vi "Write.vi"(9 "Data":u8 format="%02x", 10 "Address":u16 format="%.0x", 11 "Memory in":refnum<class "Memory.lvclass">) -> (3 "Memory out":refnum<class "Memory.lvclass">)   [LabVIEW 2021, in "Memory.lvclass"]
uses:
  Memory.lvclass
  Memory.lvclass/Memory.ctl
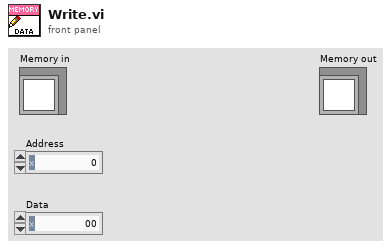
[diagram p1: front panel]
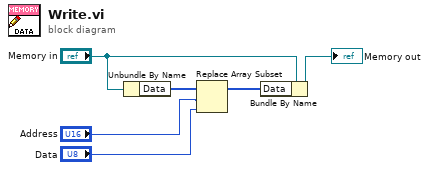
[diagram p0: block diagram]
diagram:
  n1 = Unbundle By Name("Memory in") -> ("Data"=w5:u8[])
  n2 = Replace Array Subset(array=w5, new element="Data", index="Address") -> (w4:u8[])
  n3 = Bundle By Name(cluster="Memory in", "Data"=w4) -> (→"Memory out":refnum<class "Memory.lvclass">)
